vi "Clear_Info.vi"(8 "error in (no error)":errorcluster, 9 "index in":string, 10 "buildObject":T1, 11 "IB_Source_File in":refnum<class "IB_Source_File.lvclass">) -> (0 "error out":errorcluster, 1 "index out":string, 2 "buildObject out":T1, 3 "IB_Source_File out":refnum<class "IB_Source_File.lvclass">)   [LabVIEW 2020, in "IB_Source_File.lvclass"]
uses:
  <vilib>/AppBuilder/IB_Classes/Source/File/IB_Source_File.lvclass
  <vilib>/AppBuilder/IB_Classes/Source/File/IB_Source_File.lvclass/IB_Source_File.ctl
  <vilib>/AppBuilder/IB_Classes/Source/IB_Source.lvclass
  <vilib>/AppBuilder/IB_RW_Project/IB_RW_Project_PropBag_Action.ctl
  <vilib>/AppBuilder/IB_Classes/Shortcut/IB_Shortcut.lvclass
  <resource>/Framework/Providers/API/ItemRef.ctl
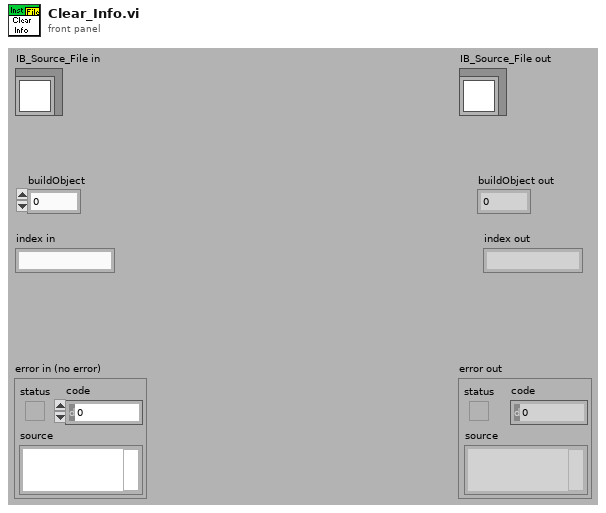
[diagram p1: front panel]
types:
  T1 = typedef "ItemRef.ctl" = u64
  T2 = typedef "IB_RW_Project_PropBag_Action.ctl" = enum16{"read", "write", "clear", "readPrevious", "writePrevious", "clearPrevious"}
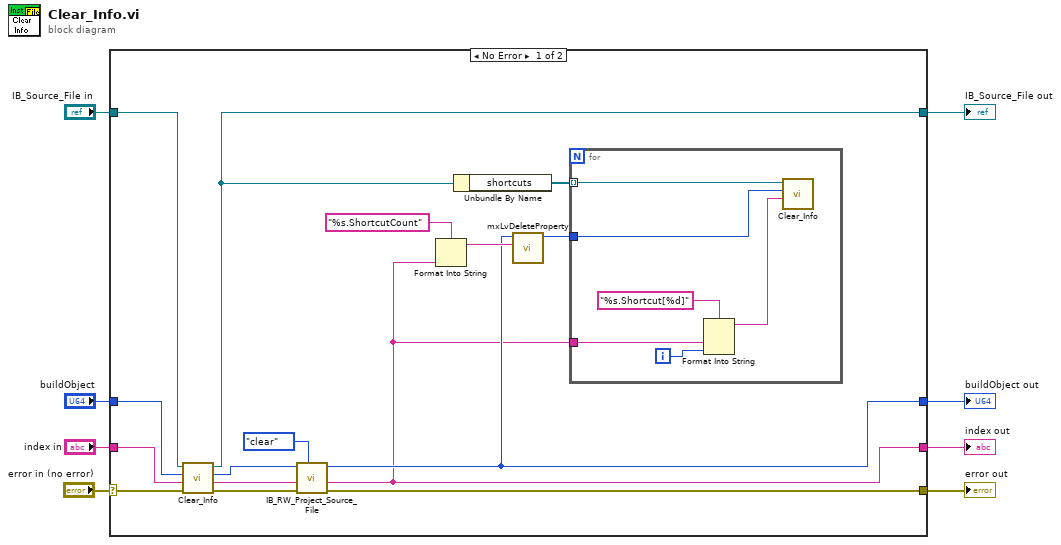
[diagram p0: block diagram]
diagram:
  n1 = case shown="No Error" "error in (no error)" {
    selector: "error in (no error)" -> [w21 w34]
    tunnel: [w18 w34] -> w8
    tunnel: [w9 w33] -> w7
    tunnel: [w11 w32] -> w6
    tunnel: [w15 w31] -> w5
    tunnel: "index in" -> [w24 w33]
    tunnel: "buildObject" -> [w23 w32]
    tunnel: "IB_Source_File in" -> [w22 w31]
    frame No Error {
      n2 = call-parent <vilib>:"Clear_Info.vi"("error in (no error)"=w21, "index in"=w24, "buildObject"=w23, "IB_Source in"=w22) -> ("error out"=w19:errorcluster, "index out"=w20:string, "buildObject out"=w17:T1, "IB_Source out"=w15:refnum<class "IB_Source_File.lvclass">)  [unwired: 4 in]
      n3 = call <vilib>:"IB_RW_Project_Source_File.vi"("action"=IB_RW_Project_PropBag_Action."clear", "error in (no error)"=w19, "index in"=w20, "buildObject"=w17) -> ("error out"=w18:errorcluster, "index out"=w9:string, "buildObject out"=w11:T1)  [unwired: 4 in, 1 out]
      n4 = Format Into String(format string="%s.ShortcutCount", w9) -> (resulting string=w12:string)  [unwired: 2 in, 1 out]
      n5 = Unbundle By Name(w15) -> ("shortcuts"=w14:refnum<class "IB_Shortcut.lvclass">[])
      n6 = call <resource>:"mxLvDeleteProperty.vi"("Tag"=w12, "Item"=w11) -> ("Item"=w10:T1)  [unwired: 1 in, 8 out]
      n7 = for {
        tunnel: w14 -> [w27] mode=indexing
        tunnel: w9 -> [w29]
        tunnel: w10 -> [w26]
        i -> [w28]
        n8 = Format Into String(format string="%s.Shortcut[%d]", w29, w28) -> (resulting string=w25:string)  [unwired: 2 in, 1 out]
        n9 = call <vilib>:"Clear_Info.vi"("index in"=w25, "buildObject"=w26, "IB_Shortcut in"=w27) -> ()  [unwired: 5 in, 4 out]
      }
    }
    frame Error {
    }
  }
  "error out" <- w8
  "IB_Source_File out" <- w5
  "buildObject out" <- w6
  "index out" <- w7
